vi "LS_372_manual_ramping.vi"(4 "Setpoint":dbl, 5 "Rate":dbl, 6 "Channel":u16, 7 "VISA-Ressourcenname":refnum<visa-resource-name>) -> ()   [LabVIEW 2019]
uses:
  Equipment/Lake Shore 372/Lake Shore 372.lvlib
panel:
  in  "Rate 2":dbl
  in  "Warmup % (50%)":dbl=50.0 min=0.0 max=100.0 step=1.0
  in  "Setpoint Change Delay (25sec)":i32=25 min=1 max=255 step=1
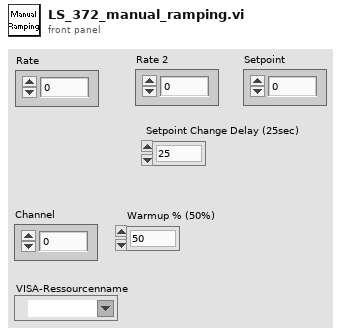
[diagram p1: front panel]
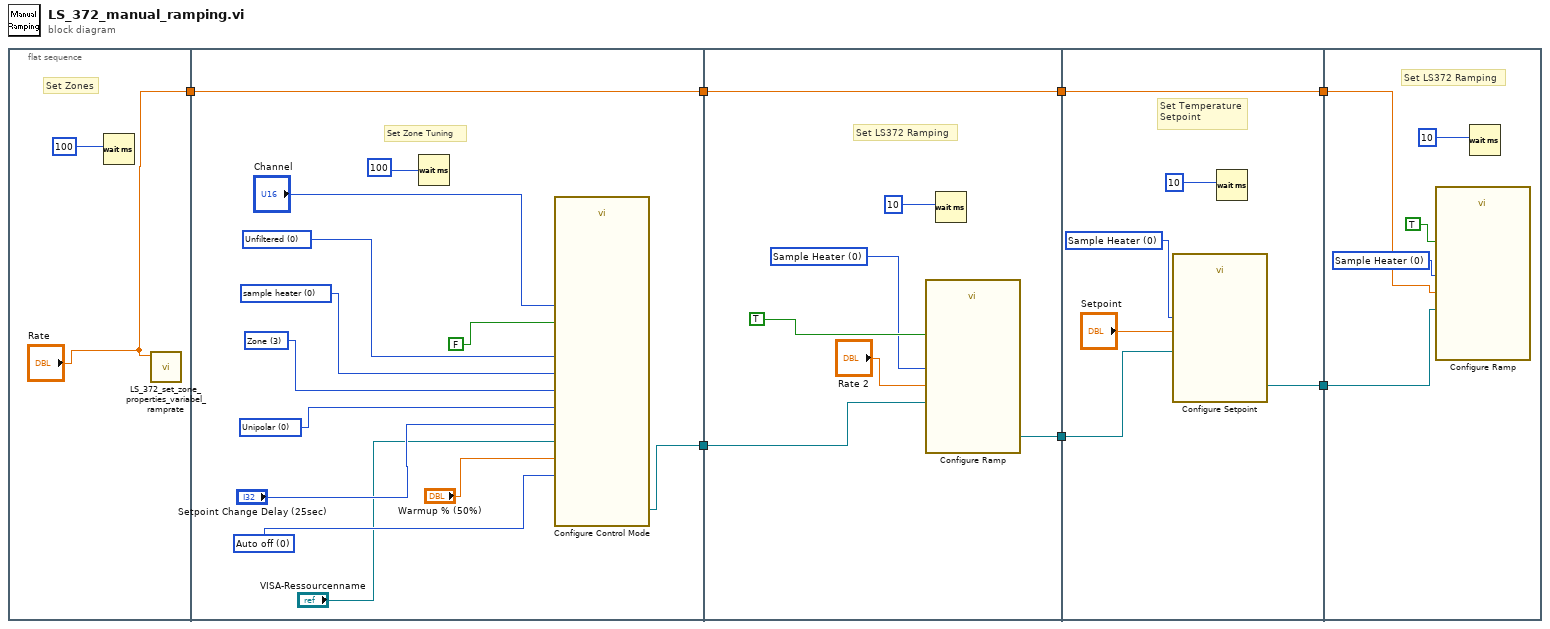
[diagram p0: block diagram]
diagram:
  n1 = flat-sequence {
    tunnel: ["Rate"] -> w2
    tunnel: [w11] -> w7
    tunnel: [w10] -> w3
    tunnel: w2 -> [w10]
    tunnel: w7 -> [w28]
    tunnel: [w24] -> w6
    tunnel: [w23] -> w4
    tunnel: w3 -> [w23]
    tunnel: w6 -> [w32]
    tunnel: [w31] -> w5
    tunnel: w4 -> [w31]
    tunnel: [w30] -> w1
    tunnel: w5 -> [w38]
    tunnel: w1 -> [w36]
    frame #0 {
      # "Set Zones"
      n2 = Wait (ms)(milliseconds to wait=100) -> ()  [unwired: 1 out]
      n3 = call "LS_372_set_zone_properties_variabel_ramprate.vi"("Ramprate"="Rate") -> ()  [unwired: 11 in]
    }
    frame #1 {
      w16 = u16 0 items=["Auto off", "Continuous"] ("Warmup Control (0: Auto off)")
      w18 = u16 0 items=["Unfiltered", "Filtered"] ("Filtered Readings (0: Unfiltered)")
      w20 = u16 0 items=["Unipolar", "Bipolar"] ("Polarity (0: Unipolar)")
      w21 = u16 0 items=["sample heater", "output 1 (warm-up heater) ", "output 2 (analog/still)"] ("Output (0: sample heater)")
      w22 = u16 3 items=["Off", "Monitor Out", "Open Loop (Manual)", "Zone", "Still", "Closed Loop (PID)", "Warm-up"] ("Output Mode (0: Off)")
      # "Set Zone Tuning"
      n4 = Wait (ms)(milliseconds to wait=100) -> ()  [unwired: 1 out]
      n5 = call "Configure Control Mode.vi"("VISA resource name"="VISA-Ressourcenname", "Enable Power-up (F: Disable)"=FALSE, "Setpoint Change Delay (25sec)"="Setpoint Change Delay (25sec)", "Output (0: sample heater)"=w21, "Channel (1:1)"="Channel", "Output Mode (0: Off)"=w22, "Polarity (0: Unipolar)"=w20, "Filtered Readings (0: Unfiltered)"=w18, "Warmup Control (0: Auto off)"=w16, "Warmup % (50%)"="Warmup % (50%)") -> ("VISA resource name out"=w11:refnum<visa-resource-name>)  [unwired: 4 in, 1 out]
    }
    frame #2 {
      w25 = u16 0 items=["Sample Heater ", "Warm-up Heater "] ("Output (0: Sample Heater)")
      # "Set LS372 Ramping"
      n6 = call "Configure Ramp.vi"("Rate Value (0.001)"="Rate 2", "Enable Ramping (F: Disable)"=TRUE, "Output (0: Sample Heater)"=w25, "VISA resource name"=w28) -> ("VISA resource name out"=w24:refnum<visa-resource-name>)  [unwired: 6 in, 1 out]
      n7 = Wait (ms)(milliseconds to wait=10) -> ()  [unwired: 1 out]
    }
    frame #3 {
      w33 = u16 0 items=["Sample Heater ", "Warm-up Heater "] ("Output (0: Sample Heater)")
      # "Set Temperature\nSetpoint"
      n8 = call "Configure Setpoint.vi"("Setpoint (0.00000E+0)"="Setpoint", "Output (0: Sample Heater)"=w33, "VISA resource name"=w32) -> ("VISA resource name out"=w30:refnum<visa-resource-name>)  [unwired: 7 in, 1 out]
      n9 = Wait (ms)(milliseconds to wait=10) -> ()  [unwired: 1 out]
    }
    frame #4 {
      w39 = u16 0 items=["Sample Heater ", "Warm-up Heater "] ("Output (0: Sample Heater)")
      # "Set LS372 Ramping"
      n10 = call "Configure Ramp.vi"("Rate Value (0.001)"=w38, "Enable Ramping (F: Disable)"=TRUE, "Output (0: Sample Heater)"=w39, "VISA resource name"=w36) -> ()  [unwired: 6 in, 2 out]
      n11 = Wait (ms)(milliseconds to wait=10) -> ()  [unwired: 1 out]
    }
  }
